vi "Teleop.vi"(10 "Match Info":T1={"Autonomous Elapsed Seconds"=0.0, "TeleOp Elapsed Seconds"=1227.288, "Disabled Elapsed Seconds"=16.859, "Visited Autonomous"=FALSE, "Visited TeleOp"=TRUE, "Visited Disabled"=TRUE, "Autonomous Settings"={"Autonomous Style"=enum."Independent", "VI Refnum"=refnum}}, 11 "Call Context":T2=enum."Stop") -> ()   [LabVIEW 2020]
doc: "This VI is called for each enabled TeleOp packet received from the DS. It is typically used to read from joysticks and other inputs and update I/O or setpoints for timed control loops. It should complete and return within 20 milliseconds or risk missing DS packets."
uses:
  <vilib>/Rock Robotics/WPI/DriverStation/WPI_DriverStationDerivedRobotMode.ctl
  <vilib>/Rock Robotics/WPI/DriverStation/WPI_DriverStationMatch Info.ctl
  <vilib>/Rock Robotics/WPI/Utilities/WPI_GetSetVariantRefNum.vi
  <vilib>/Rock Robotics/Network Tables/NT Write Boolean Array.vi
  <vilib>/Rock Robotics/Network Tables/NT Write Numeric Array.vi
panel:
  # "Cheezy Drive Settings"
  # "Enable to enable"
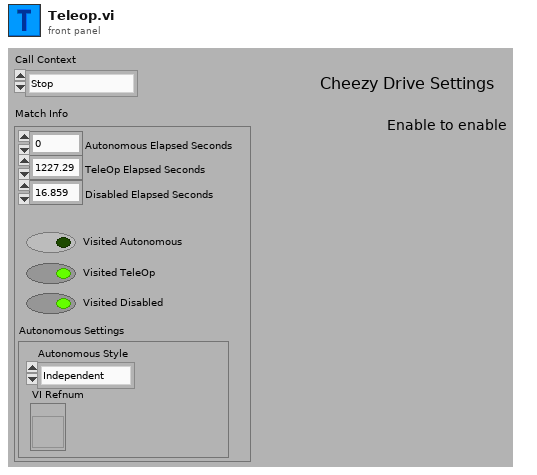
[diagram p1: front panel]
types:
  T1 = typedef "WPI_DriverStationMatch Info.ctl" = cluster{"Autonomous Elapsed Seconds":dbl, "TeleOp Elapsed Seconds":dbl, "Disabled Elapsed Seconds":dbl, "Visited Autonomous":bool, "Visited TeleOp":bool, "Visited Disabled":bool, "Autonomous Settings":cluster{"Autonomous Style":enum16{"Iterative", "Independent"}, "VI Refnum":refnum<vi>}}
  T2 = typedef "WPI_DriverStationDerivedRobotMode.ctl" = enum16{"Init", "Execute", "Stop"}
  T3 = typedef "WPI_JoystickDevRef.ctl" = cluster{"Device":T4}
  T4 = typedef "WPI_JoystickDeviceEnum.ctl" = enum16{"USB 0", "USB 1", "USB 2", "USB 3", "USB 4", "USB 5"}
  T5 = typedef "Command Status Info.ctl" = cluster{"Name":string, "Status":T6, "notifier out":T7}
  T6 = typedef "Completion Status.ctl" = enum16{"Successful", "Aborted", "Incomplete"}
  T7 = typedef "Completion Notifier.ctl" = refnum<notifier>
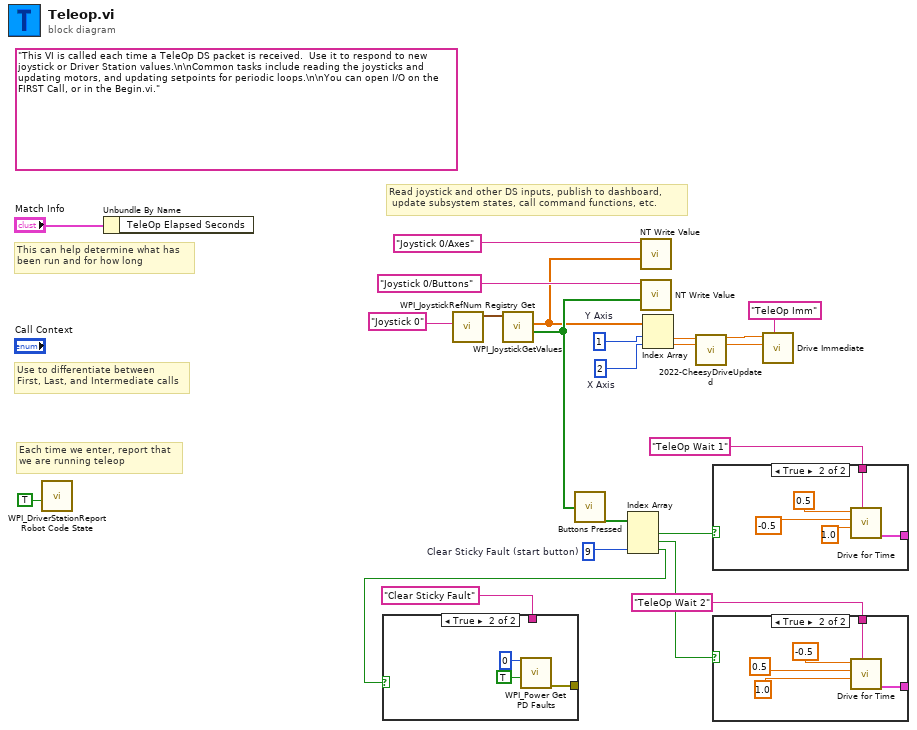
[diagram p0: block diagram]
diagram:
  w1 = 9  # Clear Sticky Fault (start button)
  w8 = 1  # Y Axis
  w7 = 2  # X Axis
  (unwired) "This VI is called each time a TeleOp DS packet is received.  Use it to respond to new joystick or Driver Station values.\n\nCommon tasks include reading the joysticks and updating motors, and updating setpoints for periodic loops.\n\nYou can open I/O on the FIRST Call, or in the Begin.vi."
  # "Read joystick and other DS inputs, publish to dashboard,\n update subsystem states, call command functions, etc."
  # "Each time we enter, report that\nwe are running teleop"
  # "Use to differentiate between\nFirst, Last, and Intermediate calls"
  # "This can help determine what has\nbeen run and for how long"
  n1 = call <vilib>:"WPI_DriverStationReport Robot Code State.vi"("TeleOp"=TRUE ("Autonomous")) -> ()  [unwired: 10 in, 1 out]
  n2 = Unbundle By Name("Match Info") -> ()  [unwired: 1 out]
  n3 = call <vilib>:"WPI_JoystickRefNum Registry Get.vi"("refnum name"="Joystick 0") -> ("JoystickDevRef"=w20:T3)  [unwired: 1 in, 9 out]
  n4 = call <vilib>:"WPI_JoystickGetValues.vi"("JoystickDevRef"=w20) -> ("Buttons"=w11:bool[], "Axes"=w10:dbl[])  [unwired: 6 in, 3 out]
  n5 = call "Buttons Pressed.vi"("Button Values"=w11) -> ("Button Presses"=w16:bool[])
  n6 = Index Array(array=w16, index #3=w1) -> (element #1=w15:bool, element #2=w14:bool, element #3=w2:bool)  [unwired: 2 in]
  n7 = case shown="True" w2 {
    tunnel: [_ w26] -> _
    tunnel: "Clear Sticky Fault" ("Description") -> [_ _]
    frame False {
    }
    frame True {
      n8 = call <vilib>:"WPI_Power Get PD Faults.vi"("Power Distribution (def)"=u8 0, "Clear Sticky Faults"=TRUE) -> ("error out"=w26:errorcluster)  [unwired: 10 in, 3 out]
    }
  }
  n9 = call-poly <vilib>:"NT Write Value.vi"("Numeric Array"=w10, "Name"="Joystick 0/Axes") -> ()  [unwired: 9 in, 1 out]
  n10 = call-poly <vilib>:"NT Write Value.vi"("Boolean Array"=w11, "Name"="Joystick 0/Buttons") -> ()  [unwired: 9 in, 1 out]
  n11 = Index Array(array=w10, index #1=w8, index #2=w7) -> (element #1=w6:dbl, element #2=w5:dbl)
  n12 = call "2022-CheesyDriveUpdated.vi"("Throttle"=w6, "Wheel"=w5) -> ("Left PWM"=w13:dbl, "Right PWM"=w4:dbl)  [unwired: 11 in, 1 out]
  n13 = case shown="True" w15 {
    tunnel: [_ w30] -> _
    tunnel: "TeleOp Wait 1" ("Description") -> [_ w29]
    frame False {
    }
    frame True {
      n14 = call "Drive for Time.vi"("Description"=w29, "Seconds"=1.0, "Right Speed"=-0.5, "Left Speed"=0.5) -> ("Command Info Out"=w30:T5)  [unwired: 7 in]
    }
  }
  n15 = case shown="True" w14 {
    tunnel: [_ w34] -> _
    tunnel: "TeleOp Wait 2" ("Description") -> [_ w33]
    frame False {
    }
    frame True {
      n16 = call "Drive for Time.vi"("Description"=w33, "Seconds"=1.0, "Right Speed"=0.5, "Left Speed"=-0.5) -> ("Command Info Out"=w34:T5)  [unwired: 7 in]
    }
  }
  n17 = call "Drive Immediate.vi"("Description"="TeleOp Imm", "Right Setpoint"=w4, "Left Setpoint"=w13) -> ()  [unwired: 8 in, 1 out]
